vi "tm_getarea_40.vi"(8 "error in (no error)":errorcluster, 11 "Handle in":u32) -> (0 "error out":errorcluster, 2 "Sub Region":T2 {"V Size"."Value" min=0 max=0 step=4; "H Size"."Value" min=0 max=0 step=4; "V Offset"."Value" min=0 max=0 step=4; "H Offset"."Value" min=0 max=0 step=4}, 3 "Handle out":u32)   [LabVIEW 2023]
uses:
  tmcamcon.dll
  <vilib>/Utility/miscctls.llb/LVMinMaxIncTypeDef.ctl
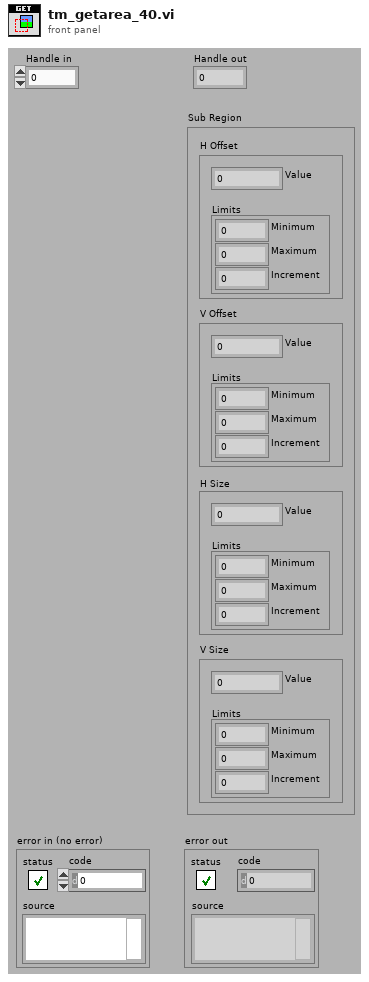
[diagram p1: front panel]
types:
  T1 = typedef "LVMinMaxIncTypeDef.ctl" = cluster{"Minimum":dbl, "Maximum":dbl, "Increment":dbl}
  T2 = cluster{"H Offset":cluster{"Value":i32, "Limits":T1}, "V Offset":cluster{"Value":i32, "Limits":T1}, "H Size":cluster{"Value":i32, "Limits":T1}, "V Size":cluster{"Value":i32, "Limits":T1}}
  T3 = cluster{"hov":i32, cluster{"hon":i32, "hox":i32, "hoi":i32}}
  T4 = cluster{"vov":i32, cluster{"von":i32, "vox":i32, "voi":i32}}
  T5 = cluster{"hwv":i32, cluster{"hwn":i32, "hwx":i32, "hwi":i32}}
  T6 = cluster{"vwv":i32, cluster{"vwn":i32, "vwx":i32, "vwi":i32}}
  T7 = cluster{cluster{"hov":i32, cluster{"hon":i32, "hox":i32, "hoi":i32}}, cluster{"vov":i32, cluster{"von":i32, "vox":i32, "voi":i32}}, cluster{"hwv":i32, cluster{"hwn":i32, "hwx":i32, "hwi":i32}}, cluster{"vwv":i32, cluster{"vwn":i32, "vwx":i32, "vwi":i32}}}
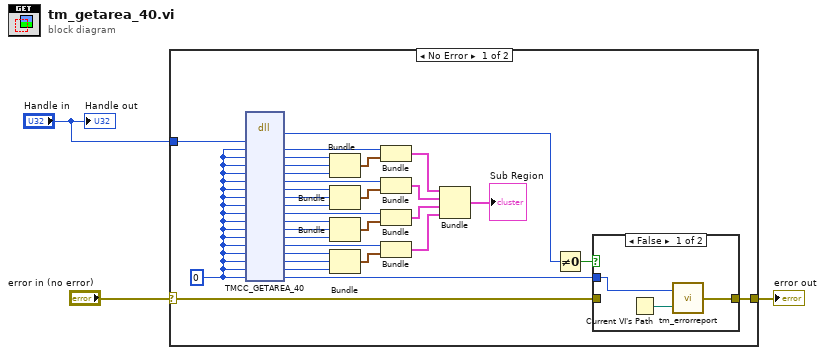
[diagram p0: block diagram]
diagram:
  n1 = case shown="No Error" "error in (no error)" {
    selector: "error in (no error)" -> [w20 w40]
    tunnel: [w17 w40] -> w2
    tunnel: "Handle in" -> [w21 _]
    frame No Error {
      w31 = 0
      n2 = dll-call lib="tmcamcon.dll" fn="TMCC_GETAREA_40"("index"=w21, "hov"=w31, "hon"=w31, "hox"=w31, "hoi"=w31, "vov"=w31, "von"=w31, "vox"=w31, "voi"=w31, "hwv"=w31, "hwn"=w31, "hwx"=w31, "hwi"=w31, "vwv"=w31, "vwn"=w31, "vwx"=w31, "vwi"=w31, "Erval"=w31) -> ("return type"=w35:u32, "hov"=w16:i32, "hon"=w33:i32, "hox"=w34:i32, "hoi"=w32:i32, "vov"=w15:i32, "von"=w30:i32, "vox"=w29:i32, "voi"=w28:i32, "hwv"=w13:i32, "hwn"=w27:i32, "hwx"=w26:i32, "hwi"=w25:i32, "vwv"=w12:i32, "vwn"=w24:i32, "vwx"=w23:i32, "vwi"=w22:i32, "Erval"=w18:i32)  [unwired: 4 in, 2 out]
      n3 = Bundle("hon"=w33, "hox"=w34, "hoi"=w32) -> (w14:cluster{"hon":i32, "hox":i32, "hoi":i32})  [unwired: 1 in]
      n4 = Bundle("von"=w30, "vox"=w29, "voi"=w28) -> (w9:cluster{"von":i32, "vox":i32, "voi":i32})  [unwired: 1 in]
      n5 = Bundle("hwn"=w27, "hwx"=w26, "hwi"=w25) -> (w10:cluster{"hwn":i32, "hwx":i32, "hwi":i32})  [unwired: 1 in]
      n6 = Bundle("vwn"=w24, "vwx"=w23, "vwi"=w22) -> (w11:cluster{"vwn":i32, "vwx":i32, "vwi":i32})  [unwired: 1 in]
      n7 = Bundle("hov"=w16, w14) -> (w8:T3)  [unwired: 1 in]
      n8 = Bundle("vov"=w15, w9) -> (w7:T4)  [unwired: 1 in]
      n9 = Bundle("hwv"=w13, w10) -> (w5:T5)  [unwired: 1 in]
      n10 = Bundle("vwv"=w12, w11) -> (w6:T6)  [unwired: 1 in]
      n11 = Bundle(w8, w7, w5, w6) -> (→"Sub Region":T7)  [unwired: 1 in]
      n12 = Not Equal To 0?(x=w35) -> (x != 0?=w19:bool)
      n13 = case shown="False" w19 {
        tunnel: w20 -> [_ w39]
        tunnel: [w37 w39] -> w17
        tunnel: w18 -> [w36 _]
        frame False {
          n14 = Current VI's Path() -> (path=w38:path)
          n15 = call "tm_errorreport.vi"("Source"=w38, "Error"=w36) -> ("error out"=w37:errorcluster)
        }
        frame True {
        }
      }
    }
    frame Error {
    }
  }
  "error out" <- w2
  "Handle out" <- "Handle in"
